vi "Drag Nodes.vi"(0 "FSM in":refnum<class "FSM.Graph.lvclass">, 9 "delta":cluster{"X":dbl, "Y":dbl}, 11 "error in (no error)":errorcluster) -> (4 "FSM out":refnum<class "FSM.Graph.lvclass">, 8 "Dragged nodes":string[](array[string]), 15 "error out":errorcluster)   [LabVIEW 2015, in "FSM.Graph.lvclass"]
uses:
  FSM.Graph.lvclass
  FSM.Graph.lvclass/FSM.Graph.ctl
  FSM.Node/FSM.Node.lvclass/FSM.Node.ctl
  FSM.Node/Read Name.vi
  FSM.Node/FSM.Node.lvclass
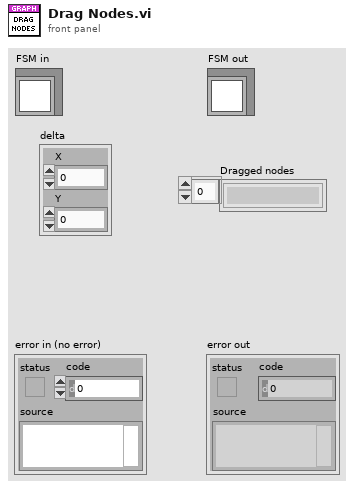
[diagram p1: front panel]
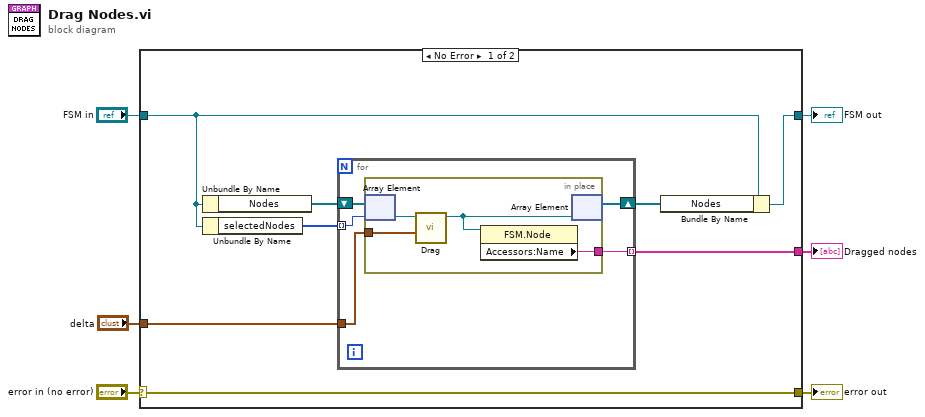
[diagram p0: block diagram]
diagram:
  n1 = case shown="No Error" "error in (no error)" {
    selector: "error in (no error)" -> [w14 w25]
    tunnel: [w14 w25] -> w5
    tunnel: [w10 w24] -> w3
    tunnel: "FSM in" -> [w13 w24]
    tunnel: "delta" -> [w7 _]
    tunnel: [w8 _] -> w1
    frame No Error {
      n2 = Unbundle By Name(w13) -> ("Nodes"=w11:refnum<class "FSM.Node.lvclass">[])
      n3 = Unbundle By Name(w13) -> ("selectedNodes"=w12:i32[])
      n4 = for {
        tunnel: w12 -> [w17] mode=indexing
        shift-right: [w16] -> w9
        shift-left: w11 -> [w18]
        tunnel: w7 -> [w19]
        tunnel: [w15] -> w8 mode=indexing
        n5 = in-place {
          in-place-border: w19 -> [w22]
          in-place-border: [w20] -> w15
          n6 = in-place-array #1(w18, w17) -> (w23:refnum<class "FSM.Node.lvclass">)
          n7 = call "Drag.vi"("delta"=w22, "FSM in"=w23) -> ("FSM out"=w21:refnum<class "FSM.Node.lvclass">)  [unwired: 8 in, 1 out]
          n8 = property class="FSM.Node"(reference=w21) -> ("Accessors:Name"=w20:string)  [unwired: 1 in, 2 out]
          n9 = in-place-array #1(w21) -> (w16:refnum<class "FSM.Node.lvclass">[])  [unwired: 1 out]
        }
      }
      n10 = Bundle By Name(cluster=w13, "Nodes"=w9) -> (w10:refnum<class "FSM.Graph.lvclass">)
    }
    frame Error {
    }
  }
  "error out" <- w5
  "FSM out" <- w3
  "Dragged nodes" <- w1
